vi "candles.vi"(11 "Array":refnum<vi>[](array[refnum])) -> ()   [LabVIEW 2014]
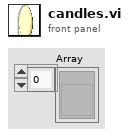
[diagram p1: front panel]
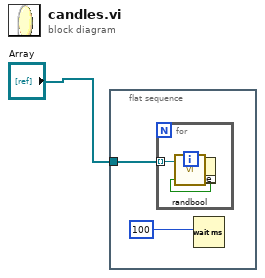
[diagram p0: block diagram]
diagram:
  n1 = flat-sequence {
    tunnel: "Array" -> [w3]
    frame #0 {
      n2 = for "For-Schleife" {
        tunnel: w3 -> [w5] mode=indexing
        n3 = call "randbool.vi"() -> ("Boolesch"=w4:bool)  [unwired: 11 in]
        n4 = property class="Bool. (strikt)"(reference=w5, "Value"=w4) -> ()  [unwired: 1 in, 2 out]
      }
      n5 = Wait (ms)(milliseconds to wait=u32 100 ("ms")) -> ()  [unwired: 1 out]
    }
  }
